vi "onHeartbeat.vi"(8 "error in (no error)":errorcluster, 10 "model in":refnum<class "IModel.lvclass">, 11 "StandbyState in":refnum<class "StandbyState.lvclass">) -> (0 "error out":errorcluster, 2 "model out":refnum<class "IModel.lvclass">, 3 "StandbyState out":refnum<class "StandbyState.lvclass">)   [LabVIEW 2016, in "States.lvlib" / "StandbyState.lvclass"]
uses:
  StandbyState.lvclass
  IModel/IModel.lvclass
  ts_sallv_sedspectrometer/DataTypes/logevent_SummaryState.ctl
  ts_sallv_sedspectrometer/SALLV_calibrationSpectrometer.lvlib
  ts_sallv_sedspectrometer/DataTypes/logevent_DetailedState.ctl
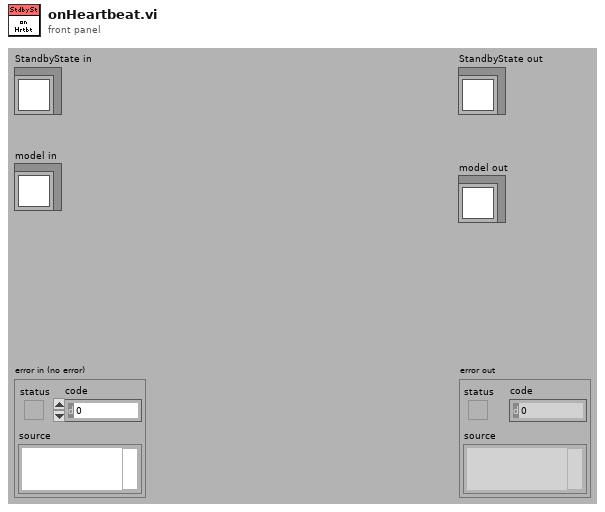
[diagram p1: front panel]
types:
  T1 = typedef "SALLV_calibrationSpectrometer.lvlib/logevent_DetailedState.ctl" = cluster{"detailedState":enum16{"", "DisabledState", "EnabledState", "FaultState", "OfflineState", "StandbyState"}, "priority":i32}
  T2 = typedef "SALLV_calibrationSpectrometer.lvlib/logevent_SummaryState.ctl" = cluster{"summaryState":enum16{"", "DisabledState", "EnabledState", "FaultState", "OfflineState", "StandbyState"}, "priority":i32}
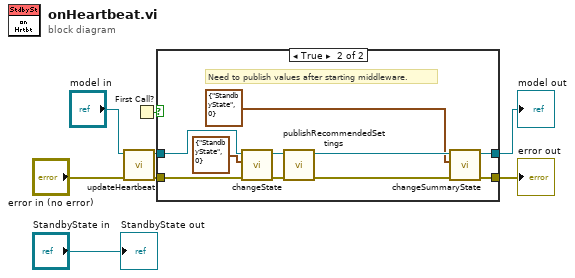
[diagram p0: block diagram]
diagram:
  n1 = call-dynamic "updateHeartbeat.vi"("error in (no error)"="error in (no error)", "IModel in"="model in") -> ("error out"=w4:errorcluster, "IModel out"=w5:refnum<class "IModel.lvclass">)  [unwired: 7 in, 1 out]
  n2 = First Call?() -> (First Call?: T/F=w1:bool)
  n3 = case shown="True" w1 {
    tunnel: w5 -> [w10 w20]
    tunnel: w4 -> [w9 w19]
    tunnel: [w10 w18] -> w3
    tunnel: [w9 w17] -> w2
    frame False {
    }
    frame True {
      # "Need to publish values after starting middleware."
      n4 = call-dynamic "changeState.vi"("error in (no error)"=w19, "DetailedState"=T1 {"detailedState"=enum."StandbyState", "priority"=0} ("logevent_DetailedState"), "IModel in"=w20) -> ("error out"=w16:errorcluster, "IModel out"=w13:refnum<class "IModel.lvclass">)  [unwired: 7 in]
      n5 = call-dynamic "publishRecommendedSettings.vi"("error in (no error)"=w16, "IModel in"=w13) -> ("error out"=w15:errorcluster, "IModel out"=w14:refnum<class "IModel.lvclass">)  [unwired: 8 in]
      n6 = call-dynamic "changeSummaryState.vi"("error in (no error)"=w15, "logevent_SummaryState"=T2 {"summaryState"=enum."StandbyState", "priority"=0}, "IModel in"=w14) -> ("error out"=w17:errorcluster, "IModel out"=w18:refnum<class "IModel.lvclass">)  [unwired: 7 in]
    }
  }
  "error out" <- w2
  "model out" <- w3
  "StandbyState out" <- "StandbyState in"
